vi "Function_SyringeSetupAssay.vi"(2 "PumpID":string="mm", 3 "Diameter (mm)":dbl, 5 "VISA resource name in":refnum<visa-resource-name>, 7 "error in":errorcluster, 8 "Direction":string(combo)="inf", 9 "Target Vol1":dbl caption="Target Vol (ul)", 10 "Units":string(combo)="mm", 11 "Set rate":dbl format="%#_4g") -> (4 "VISA resource name out":refnum<visa-resource-name>, 6 "error out":errorcluster)   [LabVIEW 2020]
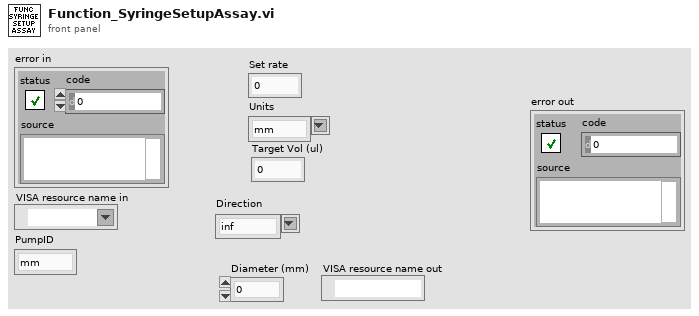
[diagram p1: front panel]
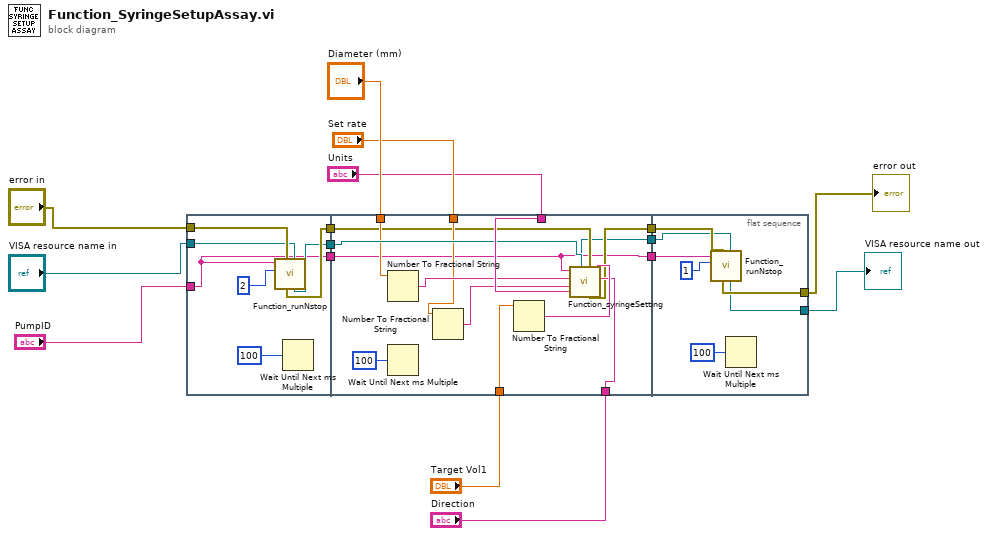
[diagram p0: block diagram]
diagram:
  n1 = flat-sequence {
    tunnel: "error in" -> [w23]
    tunnel: "VISA resource name in" -> [w22]
    tunnel: [w21] -> w16
    tunnel: [w20] -> w15
    tunnel: "PumpID" -> [w17]
    tunnel: [w17] -> w2
    tunnel: "Direction" -> [w36]
    tunnel: "Units" -> [w35]
    tunnel: "Target Vol1" -> [w34]
    tunnel: "Diameter (mm)" -> [w30]
    tunnel: "Set rate" -> [w28]
    tunnel: w16 -> [w26]
    tunnel: w15 -> [w33]
    tunnel: [w32] -> w14
    tunnel: [w25] -> w13
    tunnel: w2 -> [w24]
    tunnel: [w24] -> w1
    tunnel: w14 -> [w44]
    tunnel: w13 -> [w43]
    tunnel: [w42] -> w4
    tunnel: [w41] -> w5
    tunnel: w1 -> [w38]
    frame #0 {
      n2 = call "Function_runNstop.vi"("VISA resource name in"=w22, "error in"=w23, "condition"=2, "Server addr"=w17) -> ("VISA resource name out"=w20:refnum<visa-resource-name>, "error out"=w21:errorcluster)  [unwired: 6 in]
      n3 = Wait Until Next ms Multiple(millisecond multiple=u32 100) -> ()  [unwired: 1 out]
    }
    frame #1 {
      n4 = Number To Fractional String(number=w30) -> (F-format string=w29:string)  [unwired: 3 in]
      n5 = Wait Until Next ms Multiple(millisecond multiple=u32 100) -> ()  [unwired: 1 out]
      n6 = Number To Fractional String(number=w28) -> (F-format string=w27:string)  [unwired: 3 in]
      n7 = Number To Fractional String(number=w34) -> (F-format string=w37:string)  [unwired: 3 in]
      n8 = call "Function_syringeSetting.vi"("Direction"=w36, "target volume- string"=w37, "error in"=w26, "VISA resource name in"=w33, "units"=w35, "set rate- string"=w27, "diameter(mm)-string"=w29, "address (string)"=w24) -> ("error out"=w32:errorcluster, "VISA resource name out"=w25:refnum<visa-resource-name>)  [unwired: 2 in]
    }
    frame #2 {
      n9 = call "Function_runNstop.vi"("VISA resource name in"=w43, "error in"=w44, "condition"=1, "Server addr"=w38) -> ("VISA resource name out"=w41:refnum<visa-resource-name>, "error out"=w42:errorcluster)  [unwired: 6 in]
      n10 = Wait Until Next ms Multiple(millisecond multiple=u32 100) -> ()  [unwired: 1 out]
    }
  }
  "error out" <- w4
  "VISA resource name out" <- w5
